vi "Do i measure this quad.vi"(11 "Cell details":T1={"Measure?"=TRUE, "Area (cm^2)"=0.0, "Cell Label"="", "Cell Description"="", "Cell Position"=0, "Time in rig (s)"=0.0, "Time to next scan (s)"=0.0, "Scan number"=0.0, "When did you stick it in?"=0.0, "Time between scans (s)"=0.0, "Time of the last scan (s)"=0.0, "Scan settings in queue"=0, "Sample Holder"=0.0} {"Scan settings in queue" items=["Regular", "Inverted"]; "Time of the last scan (s)" format="%<%H:%M:%S>t"; "When did you stick it in?" format="%<%H:%M:%S>t"; "Time to next scan (s)" format="%<%H:%M:%S>t"; "Time in rig (s)" format="%<%H:%M:%S>t"}) -> (3 "Measure cell?":bool)   [LabVIEW 2011]
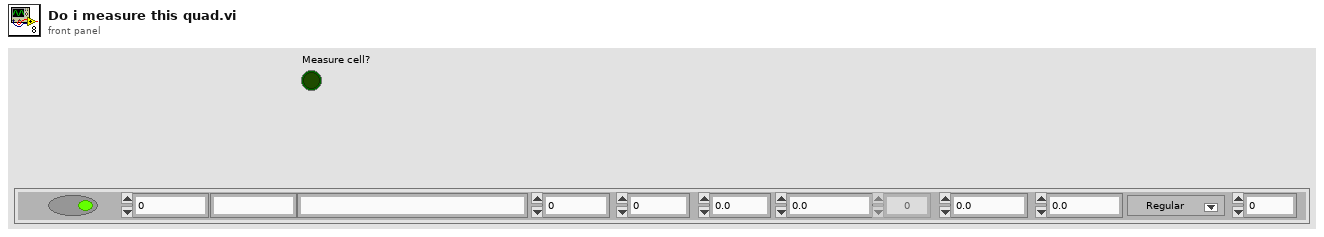
[diagram p1: front panel]
types:
  T1 = cluster{"Measure?":bool, "Area (cm^2)":dbl, "Cell Label":string, "Cell Description":string, "Cell Position":i32, "Time in rig (s)":dbl, "Time to next scan (s)":dbl, "Scan number":dbl, "When did you stick it in?":dbl, "Time between scans (s)":dbl, "Time of the last scan (s)":dbl, "Scan settings in queue":u16, "Sample Holder":dbl}
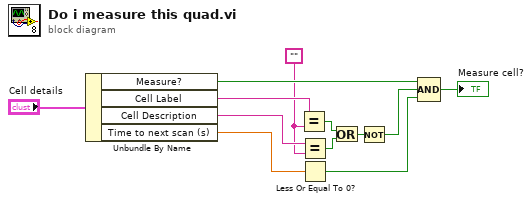
[diagram p0: block diagram]
diagram:
  w4 = ""
  n1 = Unbundle By Name("Cell details") -> ("Measure?"=w11:bool, "Cell Label"=w10:string, "Cell Description"=w9:string, "Time to next scan (s)"=w2:dbl)
  n2 = Equal?(x=w10, y=w4) -> (x = y?=w8:bool)
  n3 = Equal?(x=w9, y=w4) -> (x = y?=w7:bool)
  n4 = Less Or Equal To 0?(x=w2) -> (x <= 0?=w3:bool)
  n5 = Or(x=w8, y=w7) -> (x .or. y?=w6:bool)
  n6 = Not(x=w6) -> (.not. x?=w5:bool)
  n7 = Compound Arithmetic op=AND(w11, w5, w3) -> (→"Measure cell?":bool)
